vi "Run All.vi"(8 "Error In":errorcluster) -> (0 "Error Out":errorcluster)   [LabVIEW 2017, in "Tests.lvlib"]
uses:
  Tests.lvlib
  Support/Secret Types.ctl
  Session/Session.lvlib
  <vilib>/addons/_JKI Toolkits/Caraya/classes/Test/Test.lvclass
  KnownHosts/KnownHosts.lvlib
  KnownHost/KnownHost.lvlib
  SFTP/SFTP.lvlib
  SFTP File/SFTP File.lvlib
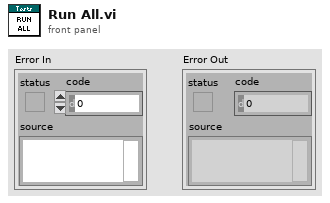
[diagram p1: front panel]
types:
  T1 = typedef "Tests.lvlib/Secret Types.ctl" = enum16{"Passphrase", "Password"}
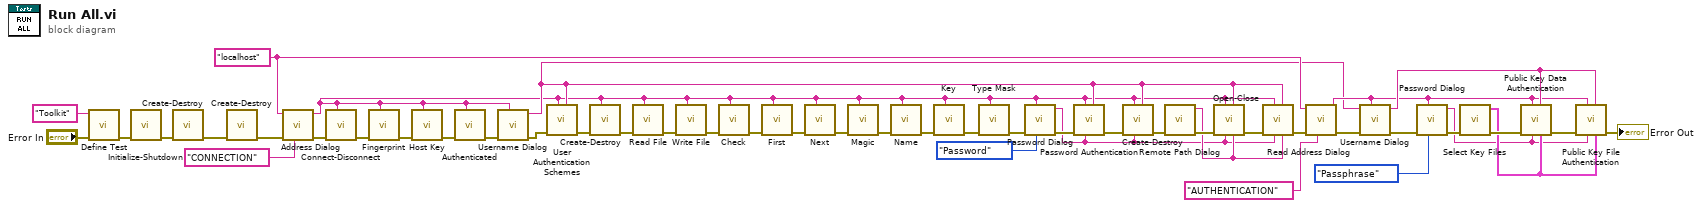
[diagram p0: block diagram]
diagram:
  w33 = "localhost" ("Address")
  n1 = call <vilib>:"Define Test.vi"("error in (no error)"="Error In", "Label (VI Title)"="Toolkit") -> ("error out"=w47:errorcluster)  [unwired: 9 in]
  n2 = call "Initialize-Shutdown.vi"("Error In"=w47) -> ("Error Out"=w48:errorcluster)  [unwired: 10 in]
  n3 = call "Create-Destroy.vi"("Error In"=w48) -> ("Error Out"=w20:errorcluster)  [unwired: 10 in]
  n4 = call "Create-Destroy.vi"("Error In"=w20) -> ("Error Out"=w25:errorcluster)  [unwired: 10 in]
  n5 = call "Address Dialog.vi"("Title"="CONNECTION", "Error In"=w25, "Address In"=w33) -> ("Error Out"=w34:errorcluster, "Address Out"=w2:string)  [unwired: 7 in]
  n6 = call "Connect-Disconnect.vi"("Address"=w2, "Error In"=w34) -> ("Error Out"=w13:errorcluster)  [unwired: 9 in]
  n7 = call "Fingerprint.vi"("Address"=w2, "Error In"=w13) -> ("Error Out"=w24:errorcluster)  [unwired: 9 in]
  n8 = call "Host Key.vi"("Address"=w2, "Error In"=w24) -> ("Error Out"=w23:errorcluster)  [unwired: 9 in]
  n9 = call "Authenticated.vi"("Address"=w2, "Error In"=w23) -> ("Error Out"=w42:errorcluster)  [unwired: 9 in]
  n10 = call "Username Dialog.vi"("Address"=w2, "Error In"=w42) -> ("Error Out"=w41:errorcluster, "Username Out"=w9:string)  [unwired: 8 in]
  n11 = call "User Authentication Schemes.vi"("Username"=w9, "Address"=w2, "Error In"=w41) -> ("Error Out"=w28:errorcluster)  [unwired: 8 in]
  n12 = call "Create-Destroy.vi"("Address"=w2, "Error In"=w28) -> ("Error Out"=w26:errorcluster)  [unwired: 9 in]
  n13 = call "Read File.vi"("Address"=w2, "Error In"=w26) -> ("Error Out"=w22:errorcluster)  [unwired: 9 in]
  n14 = call "Write File.vi"("Address"=w2, "Error In"=w22) -> ("Error Out"=w21:errorcluster)  [unwired: 9 in]
  n15 = call "Check.vi"("Address"=w2, "Error In"=w21) -> ("Error Out"=w8:errorcluster)  [unwired: 9 in]
  n16 = call "First.vi"("Address"=w2, "Error In"=w8) -> ("Error Out"=w7:errorcluster)  [unwired: 9 in]
  n17 = call "Next.vi"("Address"=w2, "Error In"=w7) -> ("Error Out"=w6:errorcluster)  [unwired: 9 in]
  n18 = call "Magic.vi"("Address"=w2, "Error In"=w6) -> ("Error Out"=w5:errorcluster)  [unwired: 9 in]
  n19 = call "Name.vi"("Address"=w2, "Error In"=w5) -> ("Error Out"=w4:errorcluster)  [unwired: 9 in]
  n20 = call "Key.vi"("Address"=w2, "Error In"=w4) -> ("Error Out"=w3:errorcluster)  [unwired: 9 in]
  n21 = call "Type Mask.vi"("Address"=w2, "Error In"=w3) -> ("Error Out"=w1:errorcluster)  [unwired: 9 in]
  n22 = call "Password Dialog.vi"("Secret Type"=Secret_Types."Password", "Address"=w2, "Error In"=w1) -> ("Error Out"=w17:errorcluster, "Password Out"=w10:string)  [unwired: 7 in]
  n23 = call "Password Authentication.vi"("Username"=w9, "Password"=w10, "Address"=w2, "Error In"=w17) -> ("Error Out"=w12:errorcluster)  [unwired: 7 in]
  n24 = call "Create-Destroy.vi"("Username"=w9, "Password"=w10, "Address"=w2, "Error In"=w12) -> ("Error Out"=w11:errorcluster)  [unwired: 7 in]
  n25 = call "Remote Path Dialog.vi"("Error In"=w11) -> ("Error Out"=w15:errorcluster, "Remote Path Out"=w14:string)  [unwired: 9 in]
  n26 = call "Open-Close.vi"("Remote Path"=w14, "Username"=w9, "Password"=w10, "Address"=w2, "Error In"=w15) -> ("Error Out"=w19:errorcluster)  [unwired: 6 in]
  n27 = call "Read.vi"("Remote Path"=w14, "Username"=w9, "Password"=w10, "Address"=w2, "Error In"=w19) -> ("Error Out"=w18:errorcluster)  [unwired: 6 in]
  n28 = call "Address Dialog.vi"("Title"="AUTHENTICATION", "Error In"=w18, "Address In"=w33) -> ("Error Out"=w37:errorcluster, "Address Out"=w32:string)  [unwired: 7 in]
  n29 = call "Username Dialog.vi"("Address"=w32, "Error In"=w37, "Username In"=w9) -> ("Error Out"=w36:errorcluster, "Username Out"=w35:string)  [unwired: 7 in]
  n30 = call "Password Dialog.vi"("Secret Type"=Secret_Types."Passphrase", "Address"=w32, "Error In"=w36) -> ("Error Out"=w39:errorcluster, "Password Out"=w38:string)  [unwired: 7 in]
  n31 = call "Select Key Files.vi"("Error In"=w39) -> ("Error Out"=w43:errorcluster, "Key Files Out"=w40:cluster{"Private":path, "Public":path})  [unwired: 9 in]
  n32 = call "Public Key Data Authentication.vi"("Key Files"=w40, "Username"=w35, "Passphrase"=w38, "Address"=w32, "Error In"=w43) -> ("Error Out"=w44:errorcluster)  [unwired: 6 in]
  n33 = call "Public Key File Authentication.vi"("Key Files"=w40, "Username"=w35, "Passphrase"=w38, "Address"=w32, "Error In"=w44) -> ("Error Out"=→"Error Out":errorcluster)  [unwired: 6 in]
